vi "erstes_graph.vi"() -> ()   [LabVIEW 2010]
panel:
  out "error out 2":errorcluster
  out "XY Graph":cluster{dbl[], dbl[]}(graph)
  out "current value":string
  in  "Wait/s":dbl format="%.2f"
  in  "Step":dbl format="%.2f"
  in  "error in (no error)":errorcluster
  in  "Stop":dbl format="%.2f"
  in  "Start":dbl format="%.2f"
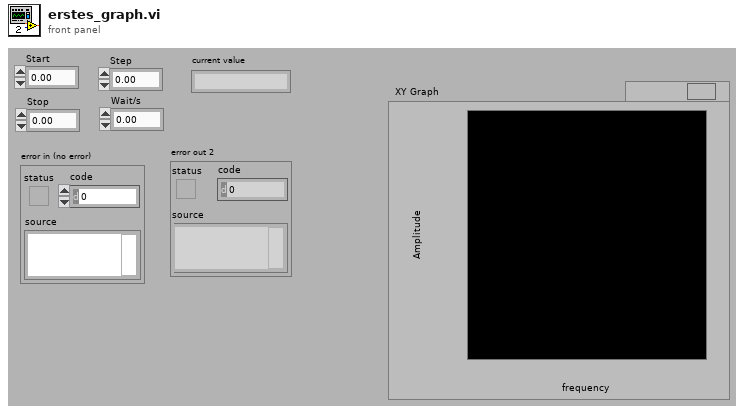
[diagram p1: front panel]
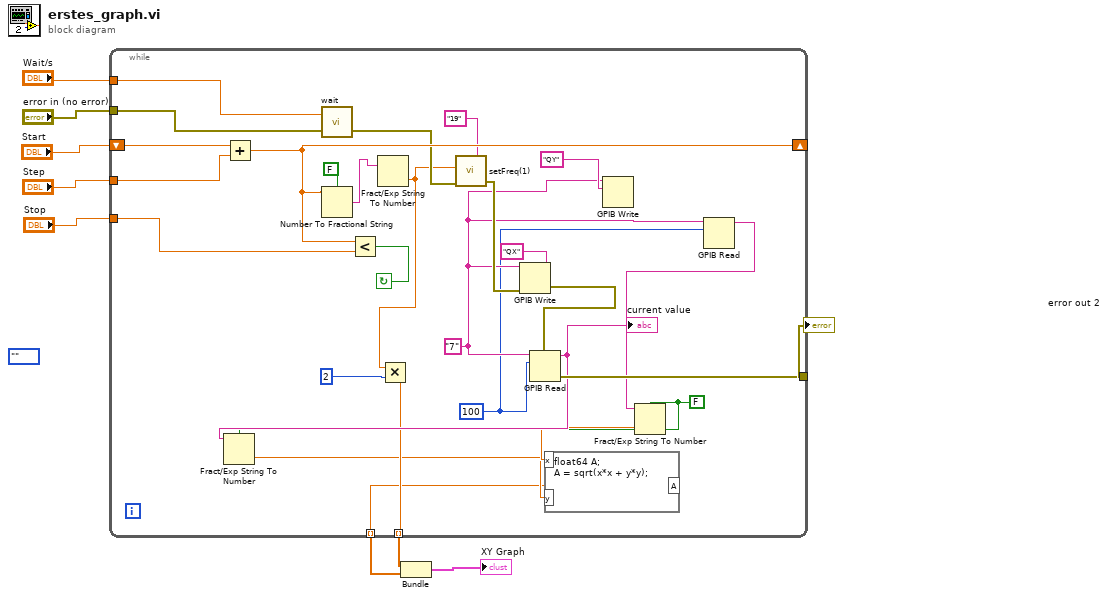
[diagram p0: block diagram]
diagram:
  (unwired) enum16{""}.""
  n1 = while {
    tunnel: "error in (no error)" -> [w28]
    shift-right: [w30] -> _
    shift-left: "Start" -> [w34]
    tunnel: "Step" -> [w36]
    tunnel: "Stop" -> [w35]
    tunnel: "Wait/s" -> [w32]
    tunnel: [w27] -> w4
    tunnel: [w12] -> w2 mode=indexing
    tunnel: [w18] -> w1 mode=indexing
    stop <- w33 continue-if-true
    w11 = FALSE
    w10 = 100
    w16 = "7"
    n2 = Add(x=w34, y=w36) -> (x+y=w30:dbl)
    n3 = call "wait.vi"("error in"=w28, "Wartezeit in Sek"=w32) -> ("error out"=w24:errorcluster)  [unwired: 1 in]
    n4 = Number To Fractional String(use system decimal point (T)=FALSE, number=w30) -> (F-format string=w22:string)  [unwired: 2 in]
    n5 = Less?(x=w30, y=w35) -> (x < y?=w33:bool)
    n6 = Fract/Exp String To Number(string=w22) -> (number=w19:dbl)  [unwired: 3 in, 1 out]
    n7 = Multiply(x=w19, y=2) -> (x*y=w18:dbl)
    n8 = call "setFreq(1).vi"("error in"=w24, "Frequenz in Hz"=w19, "address string"="19") -> ("error out"=w23:errorcluster)  [unwired: 3 in]
    n9 = GPIB Write(0:w16, 1:"QX", 3:w23) -> (6:w25:errorcluster)  [unwired: 2 in, 1 out]
    n10 = GPIB Read(0:w16, 1:w10, 3:w25) -> (5:w21:string, 7:w27:errorcluster)  [unwired: 2 in, 1 out]
    "current value" <- w21
    n11 = Fract/Exp String To Number(use system decimal point (T)=w11, string=w21) -> (number=w13:dbl)  [unwired: 2 in, 1 out]
    n12 = GPIB Write(0:w16, 1:"QY") -> ()  [unwired: 3 in, 2 out]
    n13 = GPIB Read(0:w16, 1:w10) -> (5:w15:string)  [unwired: 3 in, 2 out]
    n14 = Fract/Exp String To Number(use system decimal point (T)=w11, string=w15) -> (number=w14:dbl)  [unwired: 2 in, 1 out]
    n15 = formula code="float64 A;\nA = sqrt(x*x + y*y);"("x"=w14, "y"=w13) -> ("A"=w12:dbl)
  }
  "error out 2" <- w4
  n16 = Bundle(w1, w2) -> (→"XY Graph":cluster{dbl[], dbl[]})  [unwired: 1 in]
